vi "Execute.vi"(6 "Msg Attributes in":T1 {"Teller"."Absolute Time" format="%<%x %.3X>T"}, 7 "Actor in":refnum<class "Actor.lvclass">, 8 "Error in":errorcluster, 11 "TEMPLATE Msg in":refnum<class "TEMPLATE Msg.lvclass">) -> (0 "Error out":errorcluster, 4 "Msg Attributes out":T1 {"Teller"."Absolute Time" format="%<%x %.3X>T"}, 5 "Actor out":refnum<class "Actor.lvclass">)   [LabVIEW 2020, in "_Template.lvlib" / "Templates.lvlib" / "TEMPLATE jettl Msg.lvlib" / "TEMPLATE Msg.lvclass"]
uses:
  TEMPLATE Msg.lvclass
  TEMPLATE Msg.lvclass/TEMPLATE Msg.ctl
  TEMPLATE Msg Input/TEMPLATE Msg Input.lvclass
  TEMPLATE Msg Output/TEMPLATE Msg Output.lvclass
  jettl/jettl/Actor/Actor.lvclass
  jettl/jettl/Msg Attributes.ctl
  jettl/jettl/jettl.lvlib
  jettl/jettl/Msg Input/Msg Input.lvclass
  jettl/jettl/Msg Output/Msg Output.lvclass
  jettl/jettl/Msg/Msg.lvclass
  jettl/jettl/Teller.ctl
  jettl/jettl/Relation.ctl
panel:
  # "This front panel should not be manipulated."
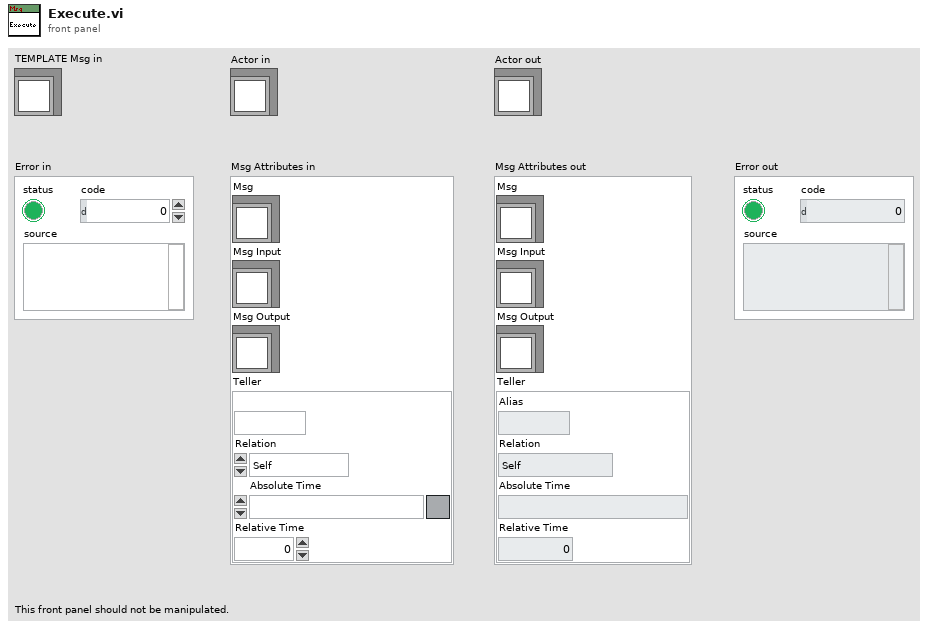
[diagram p1: front panel]
types:
  T1 = typedef "jettl.lvlib/Msg Attributes.ctl" = cluster{"Msg":refnum<class "Msg.lvclass">, "Msg Input":refnum<class "Msg Input.lvclass">, "Msg Output":refnum<class "Msg Output.lvclass">, "Teller":T2}
  T2 = typedef "jettl.lvlib/Teller.ctl" = cluster{"Alias":string, "Relation":T3, "Absolute Time":timestamp, "Relative Time":dbl}
  T3 = typedef "jettl.lvlib/Relation.ctl" = enum16{"Self", "Parent", "Child"}
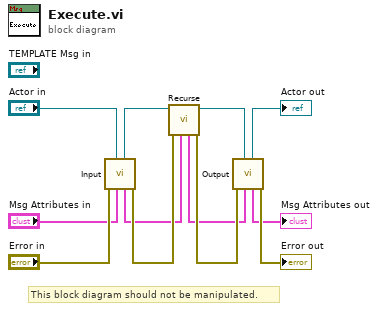
[diagram p0: block diagram]
diagram:
  # "This block diagram should not be manipulated."
  n1 = call "Input.vi"("Msg Attributes in"="Msg Attributes in", "Actor in"="Actor in", "Error in"="Error in") -> ("Error out"=w4:errorcluster, "Msg Attributes out"=w2:T1, "Actor out"=w6:refnum<class "Actor.lvclass">)  [unwired: 6 in]
  n2 = call-dynamic "Recurse.vi"("Msg Attributes in"=w2, "Error in"=w4, "Actor in"=w6) -> ("Error out"=w3:errorcluster, "Actor out"=w5:refnum<class "Actor.lvclass">, "Msg Attributes out"=w1:T1)  [unwired: 6 in]
  n3 = call "Output.vi"("Msg Attributes in"=w1, "Actor in"=w5, "Error in"=w3) -> ("Error out"=→"Error out":errorcluster, "Msg Attributes out"=→"Msg Attributes out":T1, "Actor out"=→"Actor out":refnum<class "Actor.lvclass">)  [unwired: 6 in]
